vi "Single Point Wave generation.vi"(11 "Data To Write":u16) -> (3 "error out":errorcluster)   [LabVIEW 2014]
doc: "This VI perform a single write on the DIO from 11 to 23.\nInput is a 12-bit FXP with integer part of 5-bit"
uses:
  <vilib>/rvi/eio/common/nirviEmuTemplateMethod_errors.vi
  <vilib>/eio/EIOMethodNode/EIOMethodNode.xnode
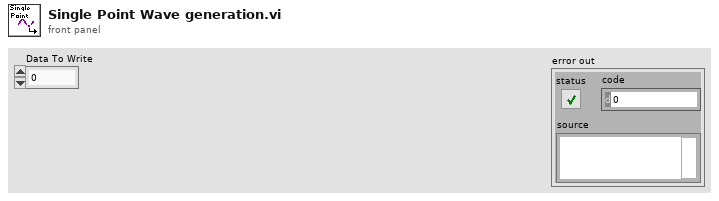
[diagram p1: front panel]
types:
  T1 = cluster{"Boolean array[0]":bool, "Boolean array[1]":bool, "Boolean array[2]":bool, "Boolean array[3]":bool, "Boolean array[4]":bool, "Boolean array[5]":bool, "Boolean array[6]":bool, "Boolean array[7]":bool, "Boolean array[8]":bool, "Boolean array[9]":bool, "Boolean array[10]":bool, "Boolean array[11]":bool}
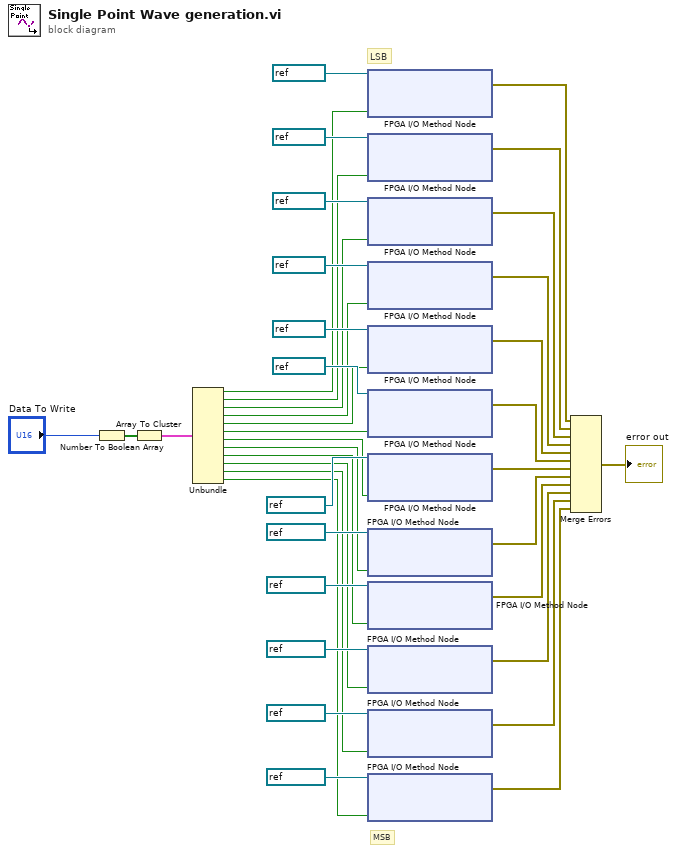
[diagram p0: block diagram]
diagram:
  # "MSB"
  # "LSB"
  n1 = Number To Boolean Array(number="Data To Write") -> (Boolean array=w28:bool[])
  n2 = Array To Cluster(array=w28) -> (cluster=w27:T1)
  n3 = Unbundle(w27) -> ("Boolean array[0]"=w26:bool, "Boolean array[1]"=w25:bool, "Boolean array[2]"=w24:bool, "Boolean array[3]"=w23:bool, "Boolean array[4]"=w22:bool, "Boolean array[5]"=w21:bool, "Boolean array[6]"=w20:bool, "Boolean array[7]"=w19:bool, "Boolean array[8]"=w18:bool, "Boolean array[9]"=w17:bool, "Boolean array[10]"=w16:bool, "Boolean array[11]"=w15:bool)
  n4 = xnode "FPGA I/O Method Node"("FPGA I/O In"=refnum<k21> "DIO4", "Data"=w26) -> ("error out"=w13:errorcluster)  [unwired: 1 in, 1 out]
  n5 = xnode "FPGA I/O Method Node"("FPGA I/O In"=refnum<k21> "DIO5", "Data"=w25) -> ("error out"=w12:errorcluster)  [unwired: 1 in, 1 out]
  n6 = xnode "FPGA I/O Method Node"("FPGA I/O In"=refnum<k21> "DIO6", "Data"=w24) -> ("error out"=w11:errorcluster)  [unwired: 1 in, 1 out]
  n7 = xnode "FPGA I/O Method Node"("FPGA I/O In"=refnum<k21> "DIO7", "Data"=w23) -> ("error out"=w10:errorcluster)  [unwired: 1 in, 1 out]
  n8 = xnode "FPGA I/O Method Node"("FPGA I/O In"=refnum<k21> "DIO8", "Data"=w22) -> ("error out"=w9:errorcluster)  [unwired: 1 in, 1 out]
  n9 = xnode "FPGA I/O Method Node"("FPGA I/O In"=refnum<k21> "DIO9", "Data"=w21) -> ("error out"=w8:errorcluster)  [unwired: 1 in, 1 out]
  n10 = xnode "FPGA I/O Method Node"("FPGA I/O In"=refnum<k21> "DIO10", "Data"=w20) -> ("error out"=w7:errorcluster)  [unwired: 1 in, 1 out]
  n11 = xnode "FPGA I/O Method Node"("FPGA I/O In"=refnum<k21> "DIO11", "Data"=w19) -> ("error out"=w6:errorcluster)  [unwired: 1 in, 1 out]
  n12 = xnode "FPGA I/O Method Node"("FPGA I/O In"=refnum<k21> "DIO12", "Data"=w18) -> ("error out"=w5:errorcluster)  [unwired: 1 in, 1 out]
  n13 = xnode "FPGA I/O Method Node"("FPGA I/O In"=refnum<k21> "DIO13", "Data"=w17) -> ("error out"=w4:errorcluster)  [unwired: 1 in, 1 out]
  n14 = xnode "FPGA I/O Method Node"("FPGA I/O In"=refnum<k21> "DIO14", "Data"=w16) -> ("error out"=w3:errorcluster)  [unwired: 1 in, 1 out]
  n15 = xnode "FPGA I/O Method Node"("FPGA I/O In"=refnum<k21> "DIO15", "Data"=w15) -> ("error out"=w2:errorcluster)  [unwired: 1 in, 1 out]
  n16 = Merge Errors(w13, w12, w11, w10, w9, w8, w7, w6, w5, w4, w3, w2) -> (→"error out":errorcluster)
